vi "Autonomous Independent.vi"   [LabVIEW 2016]
doc: "This VI is called when autonomous begins, and will automatically be terminated when autonomous ends. You can carry out timed or sensor driven robot movement independently without needing to return to the caller."
uses:
  External/External.lvlib
  <vilib>/Rock Robotics/WPI/SafetyOutput/WPI_SafetyOutputConfigMenu.ctl
types:
  T1 = typedef "WPI_SafetyOutputConfigMenu.ctl" = enum16{"Enable", "Disable"}
  T2 = typedef "WPI_RobotDriveDevRef.ctl" = cluster{"DevStatus":errorcluster, "Motors[]":T3[], "Square Inputs":bool, "Max Output":dbl}
  T3 = typedef "WPI_MotorControlDeviceRef.ctl" = cluster{"DeviceStatus":errorcluster, "Type":T4, "PWM":cluster{"PWM Channel":T5, "DeadBand":T6}, "CAN":cluster{"Device Number":u8, "SetOutput VI Ref":variant, "GetOutput VI Ref":variant, "Enable VI Ref":variant, "Disable VI Ref":variant, "Data":variant}, "Invert":bool}
  T4 = typedef "WPI_MotorControlType.ctl" = enum16{"PWM", "CAN"}
  T5 = typedef "FPGA_DIOPWMChannel.ctl" = enum8{"PWM 0", "PWM 1", "PWM 2", "PWM 3", "PWM 4", "PWM 5", "PWM 6", "PWM 7", "PWM 8", "PWM 9", "PWM MXP 0", "PWM MXP 1", "PWM MXP 2", "PWM MXP 3", "PWM MXP 4", "PWM MXP 5", "PWM MXP 6", "PWM MXP 7", "PWM MXP 8", "PWM MXP 9", "Invalid"}
  T6 = typedef "WPI_PWMDeadband.ctl" = cluster{"Name":string, "maxPositivePwm":i32, "minPositivePwm":i32, "centerPwm":i32, "maxNegativePwm":i32, "minNegativePwm":i32, "angularRange":u16}
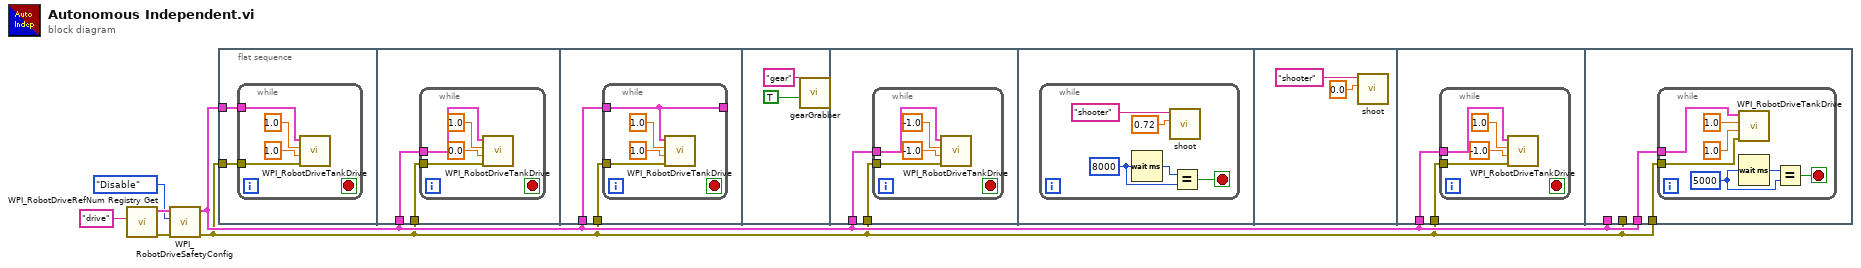
[diagram p0: block diagram]
diagram:
  n1 = call <vilib>:"WPI_RobotDriveRefNum Registry Get.vi"("refnum name"="drive") -> ("error out"=w5:errorcluster, "RobotDriveDevRef"=w4:T2)  [unwired: 9 in]
  n2 = call <vilib>:"WPI_RobotDriveSafetyConfig.vi"("error in (no error)"=w5, "mode"=WPI_SafetyOutputConfigMenu."Disable", "RobotDriveDevRef"=w4) -> ("error out"=w1:errorcluster, "RobotDriveDevRef"=w2:T2)  [unwired: 7 in]
  n3 = flat-sequence {
    tunnel: w2 -> [w8]
    tunnel: w1 -> [w7]
    tunnel: w2 -> [w14]
    tunnel: w1 -> [w13]
    tunnel: w2 -> [w20]
    tunnel: w1 -> [w19]
    tunnel: w2 -> [w28]
    tunnel: w1 -> [w27]
    tunnel: w2 -> [w41]
    tunnel: w1 -> [w40]
    tunnel: w2 -> [_]
    tunnel: w1 -> [_]
    tunnel: w2 -> [w47]
    tunnel: w1 -> [w46]
    frame #0 {
      n4 = while {
        tunnel: w8 -> [w12]
        tunnel: w7 -> [w11]
        stop <- _ stop-if-true
        n5 = call <vilib>:"WPI_RobotDriveTankDrive.vi"("error in (no error)"=w11, "Right axis value"=1.0, "Left axis value"=1.0, "RobotDriveDevRef"=w12) -> ()  [unwired: 5 in, 3 out]
      }
    }
    frame #1 {
      n6 = while {
        tunnel: w14 -> [w16]
        tunnel: w13 -> [w15]
        stop <- _ stop-if-true
        n7 = call <vilib>:"WPI_RobotDriveTankDrive.vi"("error in (no error)"=w15, "Right axis value"=0.0, "Left axis value"=1.0, "RobotDriveDevRef"=w16) -> ()  [unwired: 5 in, 3 out]
      }
    }
    frame #2 {
      n8 = while {
        tunnel: [w21] -> _
        tunnel: w19 -> [w24]
        tunnel: w20 -> [w21]
        stop <- _ stop-if-true
        n9 = call <vilib>:"WPI_RobotDriveTankDrive.vi"("error in (no error)"=w24, "Right axis value"=1.0, "Left axis value"=1.0, "RobotDriveDevRef"=w21) -> ()  [unwired: 5 in, 3 out]
      }
    }
    frame #3 {
      n10 = call "gearGrabber.vi"("gearStatus"=TRUE, "gear"="gear") -> ()  [unwired: 9 in, 1 out]
    }
    frame #4 {
      n11 = while {
        tunnel: w28 -> [w30]
        tunnel: w27 -> [w29]
        stop <- _ stop-if-true
        n12 = call <vilib>:"WPI_RobotDriveTankDrive.vi"("error in (no error)"=w29, "Right axis value"=-1.0, "Left axis value"=-1.0, "RobotDriveDevRef"=w30) -> ()  [unwired: 5 in, 3 out]
      }
    }
    frame #5 {
      n13 = while {
        stop <- w35 stop-if-true
        w36 = u32 8000 ("milliseconds to wait")
        n14 = Wait (ms)(milliseconds to wait=w36) -> (millisecond timer value=w37:u32)
        n15 = call "shoot.vi"("Motor Power"=0.72, "refnum name"="shooter") -> ()  [unwired: 9 in, 1 out]
        n16 = Equal?(x=w37, y=w36) -> (x = y?=w35:bool)
      }
    }
    frame #6 {
      n17 = call "shoot.vi"("Motor Power"=0.0, "refnum name"="shooter") -> ()  [unwired: 9 in, 1 out]
    }
    frame #7 {
      n18 = while {
        tunnel: w41 -> [w45]
        tunnel: w40 -> [w44]
        stop <- _ stop-if-true
        n19 = call <vilib>:"WPI_RobotDriveTankDrive.vi"("error in (no error)"=w44, "Right axis value"=-1.0, "Left axis value"=1.0, "RobotDriveDevRef"=w45) -> ()  [unwired: 5 in, 3 out]
      }
    }
    frame #8 {
      n20 = while {
        tunnel: w47 -> [w51]
        tunnel: w46 -> [w50]
        stop <- w52 stop-if-true
        w53 = u32 5000 ("milliseconds to wait")
        n21 = call <vilib>:"WPI_RobotDriveTankDrive.vi"("error in (no error)"=w50, "Right axis value"=1.0, "Left axis value"=1.0, "RobotDriveDevRef"=w51) -> ()  [unwired: 5 in, 3 out]
        n22 = Wait (ms)(milliseconds to wait=w53) -> (millisecond timer value=w54:u32)
        n23 = Equal?(x=w54, y=w53) -> (x = y?=w52:bool)
      }
    }
  }
